vi "Initialize.vi"(0 "VISA resource name":refnum<visa-resource-name>, 1 "ID Query (True)":bool=TRUE, 9 "Serial Configuration":T1={"Baud Rate (2400)"=2400, "Flow Control (1: XON/XOFF)"=1, "Parity (0: None)"=0, "Data Bits (7)"=7} {"Data Bits (7)" items=["7"=7, "8"=8]; "Parity (0: None)" items=["None", "Odd", "Even"]; "Flow Control (1: XON/XOFF)" items=["None", "XON/XOFF", "RTS/CTS"]; "Baud Rate (2400)" items=["600"=600, "1200"=1200, "2400"=2400, "4800"=4800, "9600"=9600, "19200"=19200]}, 11 "error in (no error)":errorcluster) -> (4 "VISA resource name out":refnum<visa-resource-name>, 15 "error out":errorcluster)   [LabVIEW 2015, in "Ohaus AV Series.lvlib"]
doc: "This VI passes the addressing information in the instrument decriptor to the Instr Open VI and returns the instrument ID. You must run this VI before using any of the instrument driver VIs for this instrument.\n\nNotes:\n\n(1) This instrument driver supports serial communication. If problems are encountered when using serial communication, it is recommended to try using baud rates less than 19,200 and hardware handshaking. \n\n(2) If you do wish to use the serial interface, set the serial settings on the instrument to be the same as the serial settings on the block diagram and in Measurement & Automation Explorer.\n\n\nIt is also important to set up the instrument so that readings can be interpreted properly.\nGoto the menu screen on the balance\n Then the PRINT-1 menu\n \n Output\n When Stable: OFF (default) \n GLP Tare: OFF (default)\n Auto Print: OFF (default)\n Content\n Number Only: OFF (default)\n Header: OFF (default)\n<B> Gross, Net, and Tare: OFF</B>\n<B> Reference: OFF</B>\n Result: ON (default)\n<B> GLP: OFF</B>\n Layout\n Line Format: MULTI (default)\n Line Feed: OFF (default)\n Form Feed: OFF (default)"
uses:
  Ohaus AV Series.lvlib
panel:
  # "(c) 2004-2009 National Instruments.  All Rights Reserved."
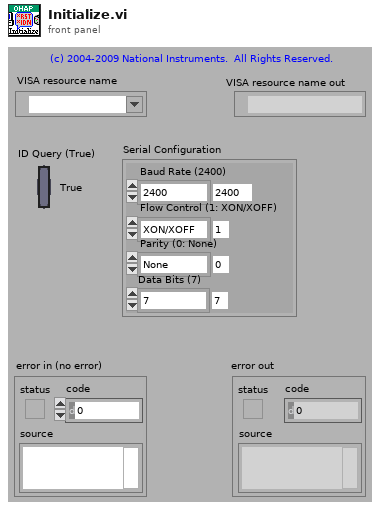
[diagram p1: front panel]
types:
  T1 = cluster{"Baud Rate (2400)":u32, "Flow Control (1: XON/XOFF)":u16, "Parity (0: None)":u16, "Data Bits (7)":u16}
  T2 = cluster{"Status":bool, "Code":i32, "Source (VI Name)":string}
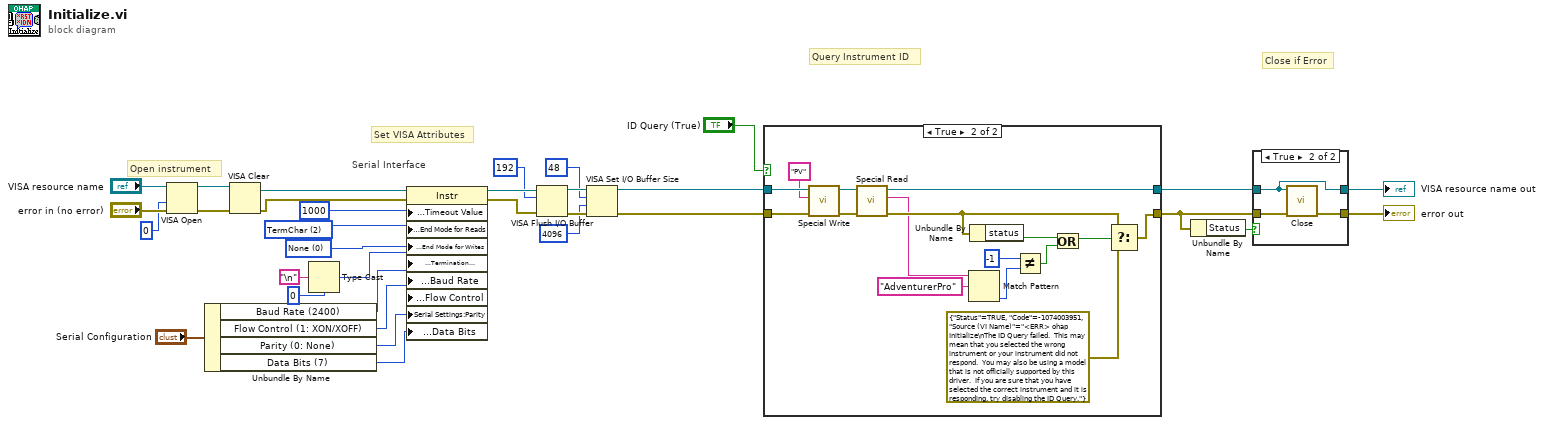
[diagram p0: block diagram]
diagram:
  w2 = u16 0 items=["None", "LastBit", "TermChar", "Break"] ("Serial Settings:Serial End Mode for Writes")
  w12 = u16 2 items=["None", "LastBit", "TermChar"] ("Serial Settings:Serial End Mode for Reads")
  # "Serial Interface"
  # "Set VISA Attributes"
  # "Close if Error"
  # "Query Instrument ID"
  # "Open instrument"
  n1 = VISA Open(access mode=u32 0, error in (no error)="error in (no error)", VISA resource name="VISA resource name") -> (VISA resource name=w28:refnum<visa-resource-name>, error out=w27:errorcluster)  [unwired: 2 in]
  n2 = Unbundle By Name("Serial Configuration") -> ("Baud Rate (2400)"=w9:u32, "Flow Control (1: XON/XOFF)"=w8:u16, "Parity (0: None)"=w6:u16, "Data Bits (7)"=w7:u16)
  n3 = VISA Clear(VISA resource name=w28, error in (no error)=w27) -> (VISA resource name out=w3:refnum<visa-resource-name>, error out=w4:errorcluster)
  n4 = Type Cast(type=u8 0, x="\n" ("Line Feed Constant")) -> (*(type *) &x=w11:u8)
  n5 = property class="Instr"(reference=w3, error in=w4, "General Settings:Timeout Value"=u32 1000, "Serial Settings:End Mode for Reads"=w12, "Serial Settings:End Mode for Writes"=w2, "Message Based Settings:Termination Character"=w11, "Serial Settings:Baud Rate"=w9, "Serial Settings:Flow Control"=w8, "Serial Settings:Parity"=w6, "Serial Settings:Data Bits"=w7) -> (reference out=w18:refnum<visa-resource-name>, error out=w20:errorcluster)
  n6 = VISA Flush I/O Buffer(VISA resource name=w18, mask (16)=u16 192, error in (no error)=w20) -> (VISA resource name out=w21:refnum<visa-resource-name>, error out=w19:errorcluster)
  n7 = VISA Set I/O Buffer Size(VISA resource name=w21, mask (16)=u16 48, size (4096)=u32 4096 ("size (0)"), error in (no error)=w19) -> (VISA resource name out=w24:refnum<visa-resource-name>, error out=w25:errorcluster)
  n8 = case shown="True" "ID Query (True)" {
    tunnel: [w34 w51] -> w22
    tunnel: [w35 w38] -> w23
    tunnel: w24 -> [w35 w41]
    tunnel: w25 -> [w34 w40]
    frame False {
    }
    frame True {
      n9 = call "Special Write.vi"("error in (no error)"=w40, "Input String"="PV" ("Write Buffer (\"\")"), "VISA resource name"=w41) -> ("error out"=w42:errorcluster, "VISA resource name out"=w37:refnum<visa-resource-name>)  [unwired: 7 in]
      n10 = call "Special Read.vi"("error in (no error)"=w42, "VISA resource name"=w37) -> ("error out"=w43:errorcluster, "Output String"=w39:string, "VISA resource name out"=w38:refnum<visa-resource-name>)  [unwired: 7 in]
      n11 = Match Pattern(string=w39, regular expression="AdventurerPro") -> (offset past match=w49:i32)  [unwired: 1 in, 3 out]
      n12 = Unbundle By Name(w43) -> ("status"=w45:bool)
      n13 = Not Equal?(x=-1, y=w49) -> (x != y?=w44:bool)
      n14 = Or(x=w45, y=w44) -> (x .or. y?=w46:bool)
      n15 = Select(t=w43, s=w46, f=T2 {"Status"=TRUE, "Code"=-1074003951, "Source (VI Name)"="<ERR> ohap Initialize\nThe ID Query failed.  This may mean that you selected the wrong instrument or your instrument did not respond.  You may also be using a model that is not officially supported by this driver.  If you are sure that you have selected the correct instrument and it is responding, try disabling the ID Query."}) -> (s? t:f=w51:T2)
    }
  }
  n16 = Unbundle By Name(w22) -> ("Status"=w26:bool)
  n17 = case shown="True" w26 {
    tunnel: w23 -> [w53 w55]
    tunnel: [w53 w55] -> w33
    tunnel: [w52 w56] -> w32
    tunnel: w22 -> [w52 w54]
    frame False {
    }
    frame True {
      n18 = call "Close.vi"("error in (no error)"=w54, "VISA resource name"=w55) -> ("error out"=w56:errorcluster)  [unwired: 9 in]
    }
  }
  "VISA resource name out" <- w33
  "error out" <- w32
